vi "Obtain Request Events.vi"(8 "error in":errorcluster, 10 "Create New? (F)":bool) -> (0 "error out":errorcluster, 2 "ATM Request Events":T1)   [LabVIEW 2020, in "ATM.lvlib"]
doc: "This VI Obtains/Creates the Requests events that will be used for other modules to communicate with the module that owns this VI. These Requests events will be accessed only via Public API methods for this module.\n\n<b>NOTE</b>: The contents of this VI are automatically generated and modified by the <b>Tools > DQMH Consortium > DQMH</b> utilities. Consider using those utilities instead of making your own modifications to this VI.\n_____\nBased on DQMH Dev Tools: Project Template 7.1.0.1503."
uses:
  ATM.lvlib
  Request Events--cluster.ctl
  Stop Argument--cluster.ctl
  Get Module Execution Status Argument--cluster.ctl
  Show Diagram Argument--cluster.ctl
  Hide Panel Argument--cluster.ctl
  Show Panel Argument--cluster.ctl
  Set Up Controls Argument--cluster.ctl
  Update ATM Messages Argument--cluster.ctl
  Start Timeout Argument--cluster.ctl
  Set Up Accounts File Argument--cluster.ctl
  Verification OK Argument--cluster.ctl
  Session Timed Out Argument--cluster.ctl
  Verification NOK Argument--cluster.ctl
  Stop Timeout Argument--cluster.ctl
  Deposit Introduced Argument--cluster.ctl
  Save Account Argument--cluster.ctl
  Check Withdrawal Argument--cluster.ctl
  Testing - Update ATM Messages Argument--cluster.ctl
  Testing - Generate File Not Found Error Argument--cluster.ctl
  Testing - Enable All Elements in FP Argument--cluster.ctl
  Testing - Disable All Elements in FP Argument--cluster.ctl
panel:
  # "NOTE: The contents of this VI are automatically generated and modified by the Tools > DQMH Consortium > DQMH utilities. Consider using those utilities instead of making your own modifications to this VI."
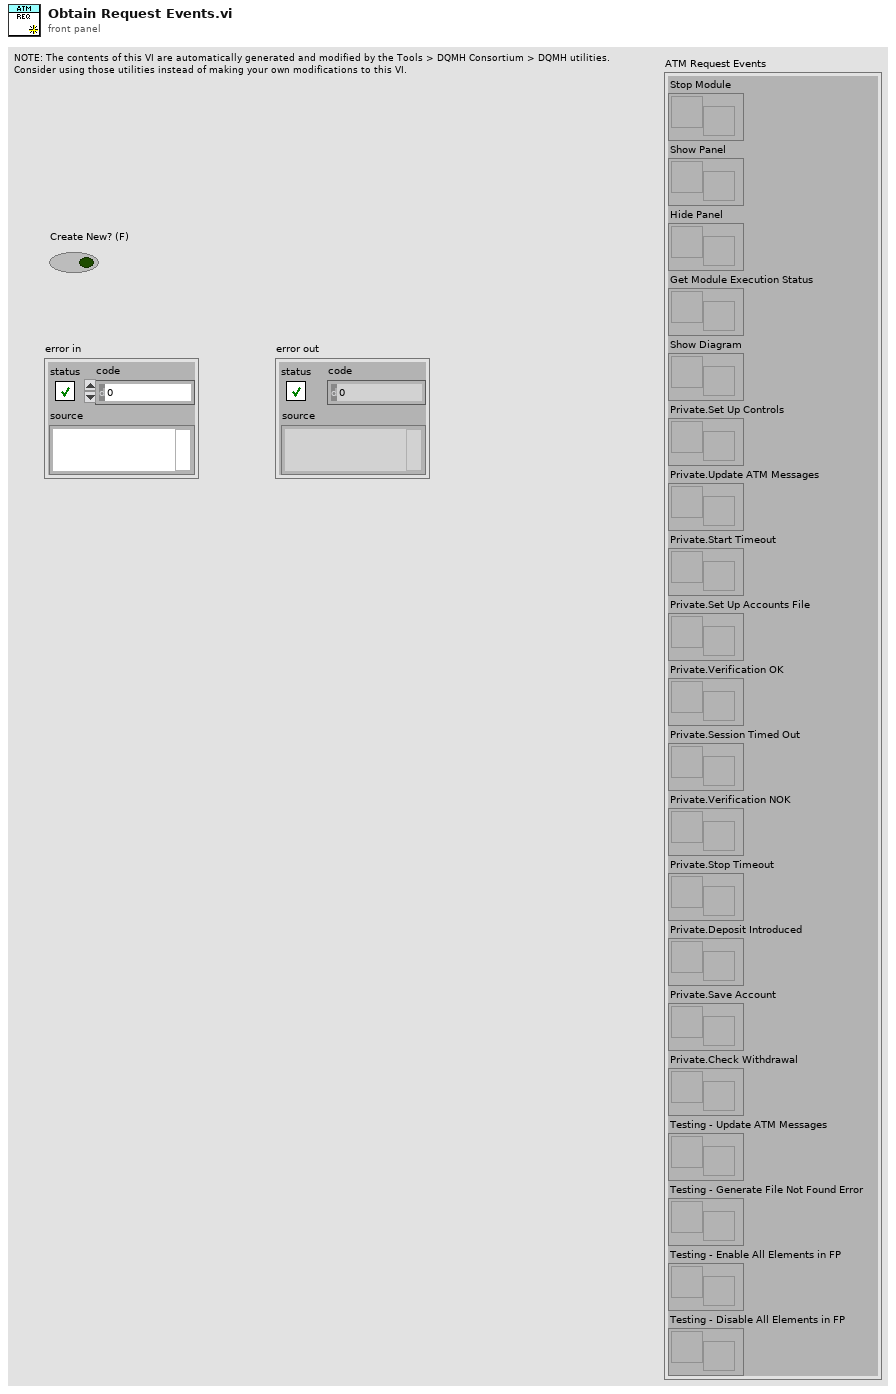
[diagram p1: front panel]
types:
  T1 = typedef "ATM.lvlib/Request Events--cluster.ctl" = cluster{"Stop Module":refnum<user-event>, "Show Panel":refnum<user-event>, "Hide Panel":refnum<user-event>, "Get Module Execution Status":refnum<user-event>, "Show Diagram":refnum<user-event>, "Private.Set Up Controls":refnum<user-event>, "Private.Update ATM Messages":refnum<user-event>, "Private.Start Timeout":refnum<user-event>, "Private.Set Up Accounts File":refnum<user-event>, "Private.Verification OK":refnum<user-event>, "Private.Session Timed Out":refnum<user-event>, "Private.Verification NOK":refnum<user-event>, "Private.Stop Timeout":refnum<user-event>, "Private.Deposit Introduced":refnum<user-event>, "Private.Save Account":refnum<user-event>, "Private.Check Withdrawal":refnum<user-event>, "Testing - Update ATM Messages":refnum<user-event>, "Testing - Generate File Not Found Error":refnum<user-event>, "Testing - Enable All Elements in FP":refnum<user-event>, "Testing - Disable All Elements in FP":refnum<user-event>}
  T2 = typedef "ATM.lvlib/Testing - Disable All Elements in FP Argument--cluster.ctl" = cluster{"Boolean":bool}
  T3 = typedef "ATM.lvlib/Testing - Enable All Elements in FP Argument--cluster.ctl" = cluster{"Boolean":bool}
  T4 = typedef "ATM.lvlib/Testing - Generate File Not Found Error Argument--cluster.ctl" = cluster{"Boolean":bool}
  T5 = typedef "ATM.lvlib/Testing - Update ATM Messages Argument--cluster.ctl" = cluster{"Boolean":bool}
  T6 = typedef "ATM.lvlib/Check Withdrawal Argument--cluster.ctl" = cluster{"Withdraw Money":i32}
  T7 = typedef "ATM.lvlib/Save Account Argument--cluster.ctl" = cluster{"Boolean":bool}
  T8 = typedef "ATM.lvlib/Deposit Introduced Argument--cluster.ctl" = cluster{"Deposit Money":u32}
  T9 = typedef "ATM.lvlib/Stop Timeout Argument--cluster.ctl" = cluster{"Boolean":bool}
  T10 = typedef "ATM.lvlib/Verification NOK Argument--cluster.ctl" = cluster{"Boolean":bool}
  T11 = typedef "ATM.lvlib/Session Timed Out Argument--cluster.ctl" = cluster{"Boolean":bool}
  T12 = typedef "ATM.lvlib/Verification OK Argument--cluster.ctl" = cluster{"Boolean":bool}
  T13 = typedef "ATM.lvlib/Set Up Accounts File Argument--cluster.ctl" = cluster{"Boolean":bool}
  T14 = typedef "ATM.lvlib/Start Timeout Argument--cluster.ctl" = cluster{"Timeout Time":i32}
  T15 = typedef "ATM.lvlib/Update ATM Messages Argument--cluster.ctl" = cluster{"ATM Messages":string}
  T16 = typedef "ATM.lvlib/Set Up Controls Argument--cluster.ctl" = cluster{"Boolean":bool}
  T17 = typedef "ATM.lvlib/Hide Panel Argument--cluster.ctl" = cluster{"Hide Panel?":bool}
  T18 = typedef "ATM.lvlib/Show Panel Argument--cluster.ctl" = cluster{"Show Panel?":bool}
  T19 = typedef "ATM.lvlib/Show Diagram Argument--cluster.ctl" = cluster{"Debug?":bool}
  T20 = typedef "ATM.lvlib/Get Module Execution Status Argument--cluster.ctl" = cluster{"Running?":bool}
  T21 = typedef "ATM.lvlib/Stop Argument--cluster.ctl" = cluster{"Origin":string, "Exit via Stop Module Req?":bool, "Wait for Module to stop?":bool}
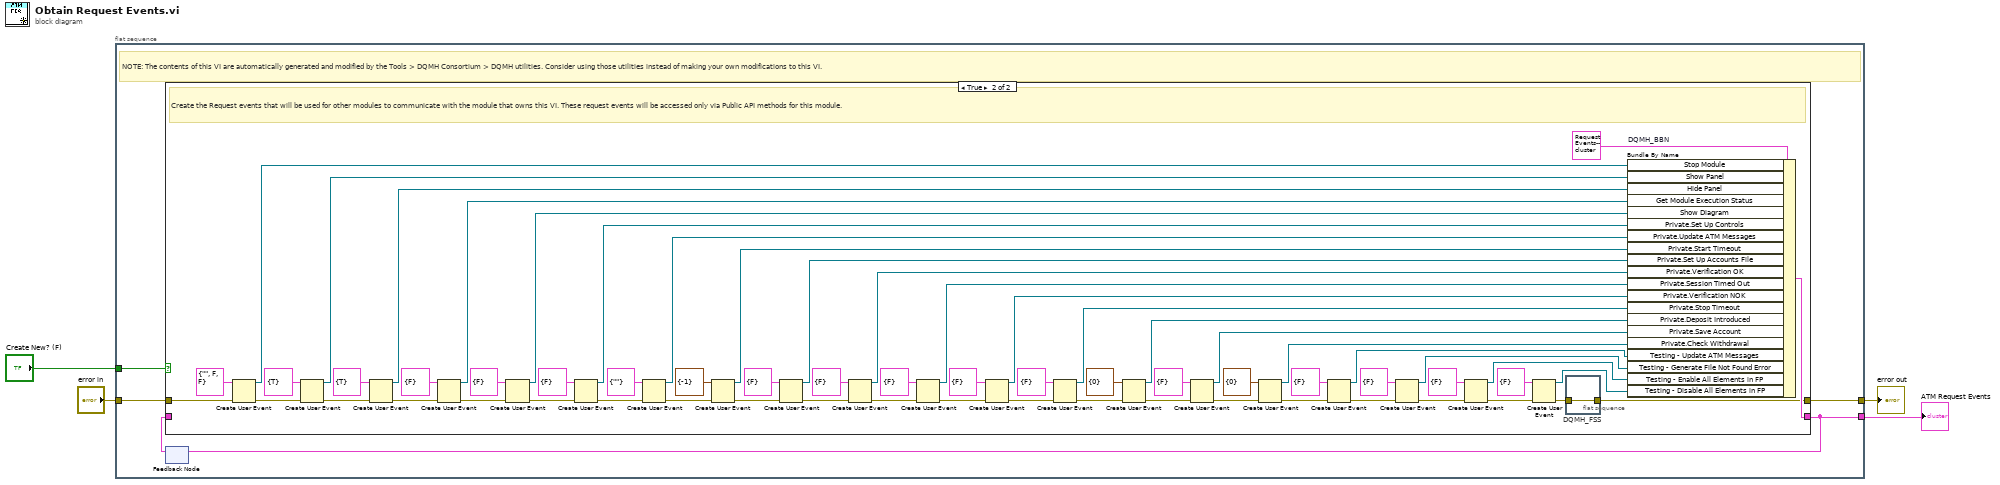
[diagram p0: block diagram]
diagram:
  n1 = flat-sequence {
    tunnel: [w9] -> w4
    tunnel: "error in" -> [w8]
    tunnel: [w6] -> w2
    tunnel: "Create New? (F)" -> [w5]
    frame #0 {
      # "NOTE: The contents of this VI are automatically generated and modified by the Tools > DQMH Consortium > DQMH utilities. Consider using those utilities instead of making your own modifications to this VI."
      n2 = feedback #1() -> (w7:T1)  [unwired: 1 in]
      n3 = case shown="True" w5 {
        tunnel: [w10 w65] -> w9
        tunnel: w8 -> [w10 w75]
        tunnel: [w11 w72] -> w6
        tunnel: w7 -> [w11 _]
        frame False {
          # "Obtain the Request events that were created in a previous call to this VI."
        }
        frame True {
          # "Create the Request events that will be used for other modules to communicate with the module that owns this VI. These request events will be accessed only via Public API methods for this module."
          n4 = Create User Event(user event datatype=T21 {"Origin"="", "Exit via Stop Module Req?"=FALSE, "Wait for Module to stop?"=FALSE} ("Stop Argument"), error in=w75) -> (user event=w73:refnum<user-event>, error out=w70:errorcluster)
          n5 = Create User Event(user event datatype=T18 {"Show Panel?"=TRUE} ("Show Panel Argument"), error in=w70) -> (user event=w69:refnum<user-event>, error out=w68:errorcluster)
          n6 = Create User Event(user event datatype=T17 {"Hide Panel?"=TRUE} ("Hide Panel Argument"), error in=w68) -> (user event=w67:refnum<user-event>, error out=w66:errorcluster)
          n7 = Create User Event(user event datatype=T20 {"Running?"=FALSE} ("Get Module Execution Status Argument"), error in=w66) -> (user event=w63:refnum<user-event>, error out=w64:errorcluster)
          n8 = Create User Event(user event datatype=T19 {"Debug?"=FALSE} ("Show Diagram Argument"), error in=w64) -> (user event=w60:refnum<user-event>, error out=w61:errorcluster)
          n9 = Create User Event(user event datatype=T16 {"Boolean"=FALSE} ("Set Up Controls Argument"), error in=w61) -> (user event=w55:refnum<user-event>, error out=w56:errorcluster)
          n10 = Create User Event(user event datatype=T15 {"ATM Messages"=""} ("Update ATM Messages Argument"), error in=w56) -> (user event=w52:refnum<user-event>, error out=w53:errorcluster)
          n11 = Create User Event(user event datatype=T14 {"Timeout Time"=-1} ("Start Timeout Argument"), error in=w53) -> (user event=w49:refnum<user-event>, error out=w50:errorcluster)
          n12 = Create User Event(user event datatype=T13 {"Boolean"=FALSE} ("Set Up Accounts File Argument"), error in=w50) -> (user event=w46:refnum<user-event>, error out=w47:errorcluster)
          n13 = Create User Event(user event datatype=T12 {"Boolean"=FALSE} ("Verification OK Argument"), error in=w47) -> (user event=w43:refnum<user-event>, error out=w44:errorcluster)
          n14 = Create User Event(user event datatype=T11 {"Boolean"=FALSE} ("Session Timed Out Argument"), error in=w44) -> (user event=w40:refnum<user-event>, error out=w41:errorcluster)
          n15 = Create User Event(user event datatype=T10 {"Boolean"=FALSE} ("Verification NOK Argument"), error in=w41) -> (user event=w37:refnum<user-event>, error out=w38:errorcluster)
          n16 = Create User Event(user event datatype=T9 {"Boolean"=FALSE} ("Stop Timeout Argument"), error in=w38) -> (user event=w34:refnum<user-event>, error out=w35:errorcluster)
          n17 = Create User Event(user event datatype=T8 {"Deposit Money"=0} ("Deposit Introduced Argument"), error in=w35) -> (user event=w31:refnum<user-event>, error out=w32:errorcluster)
          n18 = Create User Event(user event datatype=T7 {"Boolean"=FALSE} ("Save Account Argument"), error in=w32) -> (user event=w28:refnum<user-event>, error out=w29:errorcluster)
          n19 = Create User Event(user event datatype=T6 {"Withdraw Money"=0} ("Check Withdrawal Argument"), error in=w29) -> (user event=w25:refnum<user-event>, error out=w26:errorcluster)
          n20 = Create User Event(user event datatype=T5 {"Boolean"=FALSE} ("Testing - Update ATM Messages Argument"), error in=w26) -> (user event=w22:refnum<user-event>, error out=w23:errorcluster)
          n21 = Create User Event(user event datatype=T4 {"Boolean"=FALSE} ("Testing - Generate File Not Found Error Argument"), error in=w23) -> (user event=w19:refnum<user-event>, error out=w20:errorcluster)
          n22 = Create User Event(user event datatype=T3 {"Boolean"=FALSE} ("Testing - Enable All Elements in FP Argument"), error in=w20) -> (user event=w16:refnum<user-event>, error out=w17:errorcluster)
          n23 = Create User Event(user event datatype=T2 {"Boolean"=FALSE} ("Testing - Disable All Elements in FP Argument"), error in=w17) -> (user event=w13:refnum<user-event>, error out=w14:errorcluster)
          n24 = flat-sequence "DQMH_FSS" {
            tunnel: w14 -> [w76]
            tunnel: [w76] -> w65
            frame #0 {
            }
          }
          n25 = Bundle By Name "DQMH_BBN"(cluster=T1 {"Stop Module"=refnum, "Show Panel"=refnum, "Hide Panel"=refnum, "Get Module Execution Status"=refnum, "Show Diagram"=refnum, "Private.Set Up Controls"=refnum, "Private.Update ATM Messages"=refnum, "Private.Start Timeout"=refnum, "Private.Set Up Accounts File"=refnum, "Private.Verification OK"=refnum, "Private.Session Timed Out"=refnum, "Private.Verification NOK"=refnum, "Private.Stop Timeout"=refnum, "Private.Deposit Introduced"=refnum, "Private.Save Account"=refnum, "Private.Check Withdrawal"=refnum, "Testing - Update ATM Messages"=refnum, "Testing - Generate File Not Found Error"=refnum, "Testing - Enable All Elements in FP"=refnum, "Testing - Disable All Elements in FP"=refnum} ("output cluster"), "Stop Module"=w73, "Show Panel"=w69, "Hide Panel"=w67, "Get Module Execution Status"=w63, "Show Diagram"=w60, "Private.Set Up Controls"=w55, "Private.Update ATM Messages"=w52, "Private.Start Timeout"=w49, "Private.Set Up Accounts File"=w46, "Private.Verification OK"=w43, "Private.Session Timed Out"=w40, "Private.Verification NOK"=w37, "Private.Stop Timeout"=w34, "Private.Deposit Introduced"=w31, "Private.Save Account"=w28, "Private.Check Withdrawal"=w25, "Testing - Update ATM Messages"=w22, "Testing - Generate File Not Found Error"=w19, "Testing - Enable All Elements in FP"=w16, "Testing - Disable All Elements in FP"=w13) -> (w72:T1)
        }
      }
      n26 = feedback-in #1(w6) -> ()
    }
  }
  "ATM Request Events" <- w2
  "error out" <- w4
